vi "Create Cursor Point.vi"(5 "Cursor Point":T1, 6 "Scale":T4, 7 "Cursor Position":T3, 8 "error in (no error)":errorcluster, 9 "Cursor ID":i32, 11 "Cursor Object In":refnum<vi>) -> (0 "error out":errorcluster, 3 "Cursor Object Out":refnum<vi>)   [LabVIEW 2020, in "3D Plot.lvclass"]
uses:
  3D Plot.lvclass
  Cursor Point.ctl
  Sprite Type.ctl
  NI_3D Picture Control.lvlib
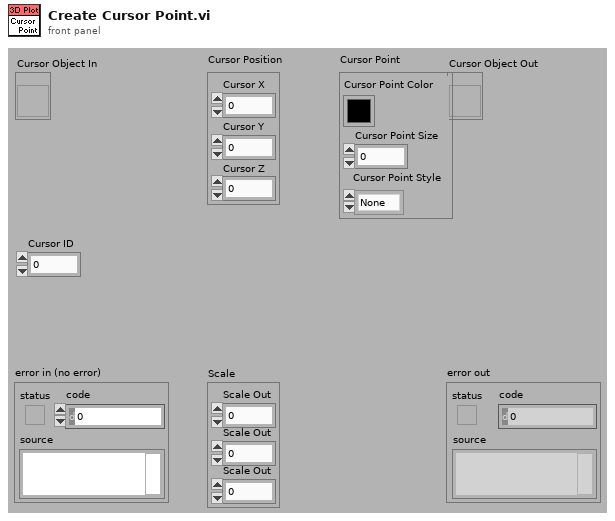
[diagram p1: front panel]
types:
  T1 = typedef "3D Plot.lvclass/Cursor Point.ctl" = cluster{"Cursor Point Color":u32, "Cursor Point Size":sgl, "Cursor Point Style":T2}
  T2 = typedef "3D Plot.lvclass/Sprite Type.ctl" = enum16{"None", "Empty Square", "Solid Square", "Empty Diamond", "Solid Diamond", "Empty Circle", "Solid Circle", "Asterisk", "Bold X", "Wireframe Sphere", "Solid Sphere", "Wireframe Cube", "Solid Cube"}
  T3 = cluster{"Cursor X":sgl, "Cursor Y":sgl, "Cursor Z":sgl}
  T4 = cluster{"Scale Out":sgl, "Scale Out":sgl, "Scale Out":sgl}
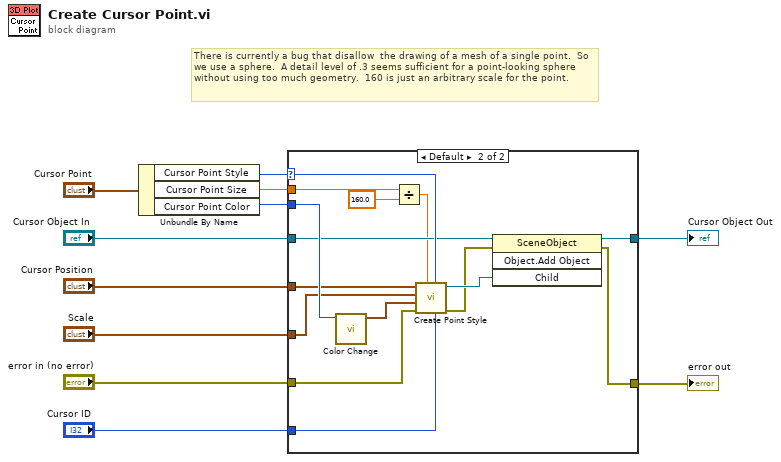
[diagram p0: block diagram]
diagram:
  # "There is currently a bug that disallow  the drawing of a mesh of a single point.  So we use a sphere.  A detail level of .3 seems sufficient for a point-looking sphere without using too much geometry.  160 is just an arbitrary scale for the point."
  n1 = Unbundle By Name("Cursor Point") -> ("Cursor Point Style"=w4:T2, "Cursor Point Size"=w3:sgl, "Cursor Point Color"=w2:u32)
  n2 = case shown="Default" w4 {
    selector: w4 -> [_ w27]
    tunnel: "Cursor Position" -> [_ w26]
    tunnel: w2 -> [_ w28]
    tunnel: "Cursor Object In" -> [w13 w22]
    tunnel: w3 -> [_ w18]
    tunnel: [w13 w21] -> w11
    tunnel: "Scale" -> [_ w24]
    tunnel: "error in (no error)" -> [w12 w23]
    tunnel: [w12 w20] -> w8
    tunnel: "Cursor ID" -> [_ w14]
    frame "None" {
    }
    frame Default {
      n3 = call "Color Change.vi"("Color"=w28) -> ("RGBA"=w25:cluster{"R":sgl, "G":sgl, "B":sgl, "A":sgl})  [unwired: 1 in, 9 out]
      n4 = Divide(x=w18, y=sgl 160.0) -> (x/y=w17:sgl)
      n5 = call "Create Point Style.vi"("Cursor ID"=w14, "Sprite Type"=w27, "Size"=w17, "error in (no error)"=w23, "RGBA"=w25, "Scale"=w24, "Position"=w26) -> ("error out"=w15:errorcluster, "Scene:New Object"=w16:refnum<vi>)  [unwired: 1 in, 2 out]
      n6 = invoke class="SceneObject" method="Object.Add Object"(reference=w22, error in=w15, "Child"=w16) -> (reference out=w21:refnum<vi>, error out=w20:errorcluster)  [unwired: 1 in, 2 out]
    }
  }
  "Cursor Object Out" <- w11
  "error out" <- w8
